vi "Check Write Size.vi"(8 "error in (no error)":errorcluster, 10 "# Of Waveforms":i32, 11 "Waveform Session in":refnum<class "Waveform Session.lvclass">) -> (0 "error out":errorcluster, 3 "Waveform Session out":refnum<class "Waveform Session.lvclass">)   [LabVIEW 2020, in "NI_VS Custom Device Waveform API.lvlib" / "Waveform Session.lvclass"]
uses:
  Waveform Session.lvclass
  Waveform Session.lvclass/Waveform Session.ctl
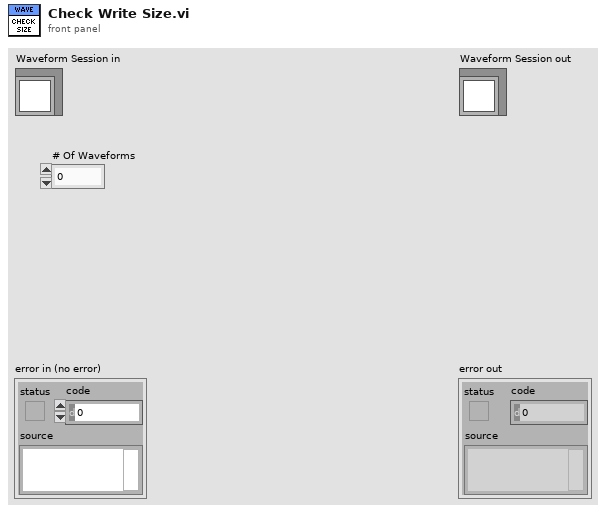
[diagram p1: front panel]
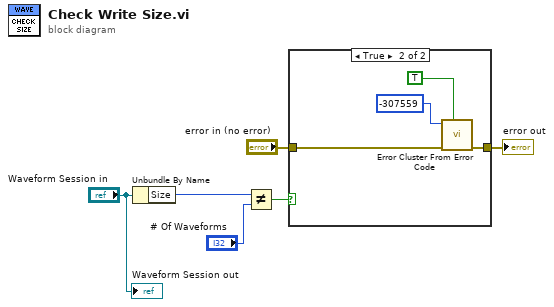
[diagram p0: block diagram]
diagram:
  n1 = Unbundle By Name("Waveform Session in") -> ("Size"=w4:i32)
  n2 = Not Equal?(x=w4, y="# Of Waveforms") -> (x != y?=w3:bool)
  n3 = case shown="True" w3 {
    tunnel: "error in (no error)" -> [w7 w11]
    tunnel: [w7 w9] -> w2
    frame False {
    }
    frame True {
      n4 = call <vilib>:"Error Cluster From Error Code.vi"("show call chain? (False)"=TRUE, "error in (no error)"=w11, "error code (0)"=-307559) -> ("error out"=w9:errorcluster)  [unwired: 6 in]
    }
  }
  "error out" <- w2
  "Waveform Session out" <- "Waveform Session in"
